vi "Open My Data CSV.vi"(5 "Comment":string, 7 "Time Stamp":timestamp, 8 "error in":errorcluster, 11 "file path":path) -> (0 "error out":errorcluster, 3 "refnum out":refnum<file>)   [LabVIEW 2014]
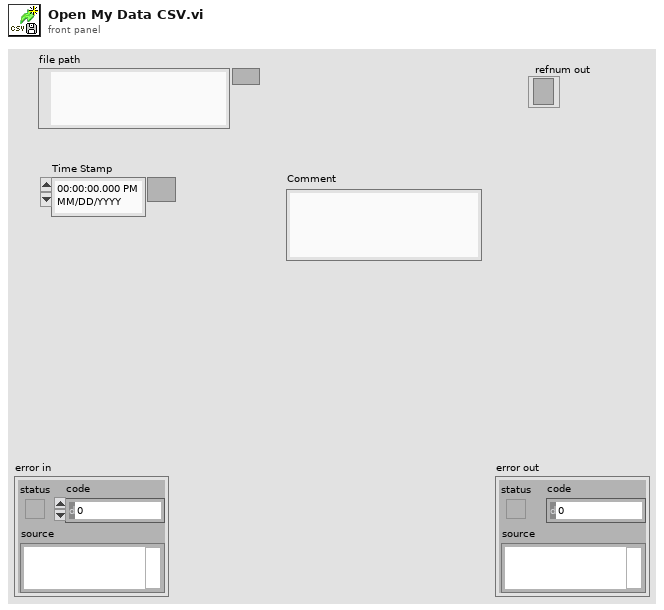
[diagram p1: front panel]
types:
  T1 = enum16{"open", "replace", "create", "open or create", "replace or create", "replace or create with confirmation"}
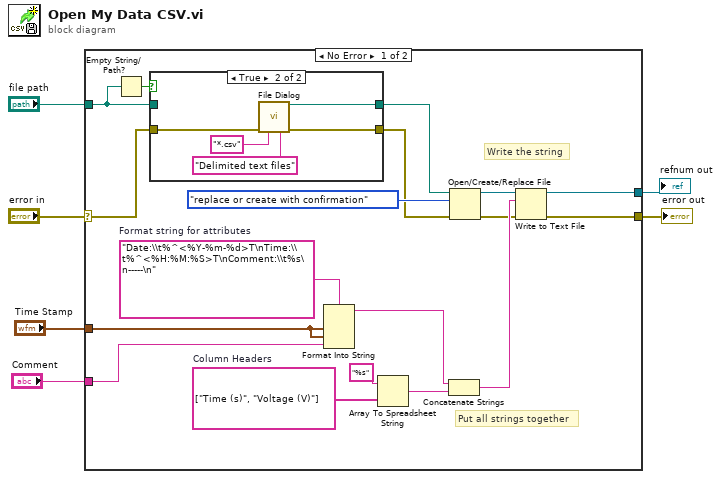
[diagram p0: block diagram]
diagram:
  n1 = case shown="No Error" "error in" {
    selector: "error in" -> [w10 w32]
    tunnel: [w20 w32] -> w6
    tunnel: "file path" -> [w7 _]
    tunnel: "Time Stamp" -> [w18 _]
    tunnel: "Comment" -> [w17 _]
    tunnel: [w15 _] -> w1
    frame No Error {
      w19 = "Date:\\t%^<%Y-%m-%d>T\nTime:\\t%^<%H:%M:%S>T\nComment:\\t%s\n-----\n"  # Format string for attributes
      w24 = string[] ["Time (s)", "Voltage (V)"]  # Column Headers
      # "Write the string"
      # "Put all strings together"
      n2 = Empty String/Path?(string/path=w7) -> (empty?=w11:bool)
      n3 = case shown="True" w11 {
        tunnel: w10 -> [w25 w29]
        tunnel: [w25 w28] -> w9
        tunnel: [w26 w27] -> w8
        tunnel: w7 -> [w26 _]
        frame False {
        }
        frame True {
          n4 = call "File Dialog"("error in"=w29, "pattern (all files)"="*.csv", "pattern label"="Delimited text files") -> ("selected path"=w27:path, "error out"=w28:errorcluster)  [unwired: 9 in, 2 out]
        }
      }
      n5 = Format Into String(format string=w19, w18, w18, w17) -> (resulting string=w16:string)  [unwired: 2 in, 1 out]
      n6 = Array To Spreadsheet String(array=w24, 3:"%s" ("format string")) -> (spreadsheet string=w23:string)  [unwired: 1 in]
      n7 = Concatenate Strings(w16, w23) -> (w22:string)
      n8 = Open/Create/Replace File(file path (use dialog)=w8, error in=w9, operation (0:open)=T1."replace or create with confirmation") -> (refnum out=w14:refnum<file>, error out=w13:errorcluster)  [unwired: 3 in, 1 out]
      n9 = Write to Text File(file (use dialog)=w14, text=w22, error in=w13) -> (refnum out=w15:refnum<file>, error out=w20:errorcluster)  [unwired: 1 in, 1 out]
    }
    frame Error {
      # "Wire previous error through"
    }
  }
  "error out" <- w6
  "refnum out" <- w1
